vi "01.vi"() -> ()   [LabVIEW 2015]
uses:
  Libraries/LibSDL2 Wrapper/Controls/Init Flags.ctl
  Libraries/LibSDL2 Wrapper/LibSDL2.lvlib
panel:
  out "Error":string
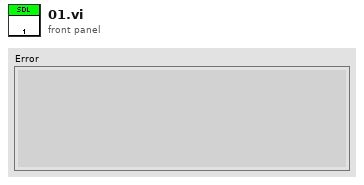
[diagram p1: front panel]
types:
  T1 = typedef "LibSDL2.lvlib/Init Flags.ctl" = u32
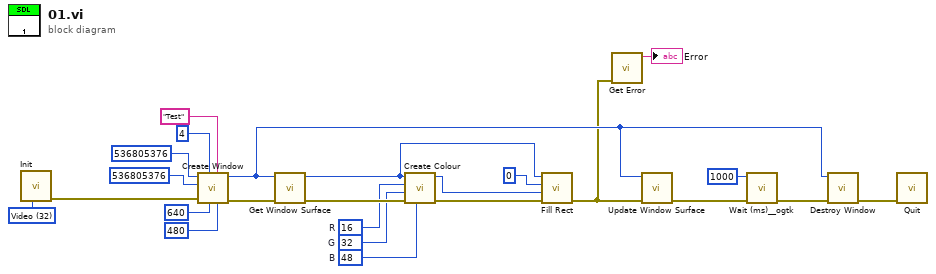
[diagram p0: block diagram]
diagram:
  w1 = u8 48  # B
  w2 = u8 32  # G
  w5 = u8 16  # R
  w24 = T1 32 items=["Timer"=1, "Audio"=16, "Video"=32, "Joystick"=512, "Haptic"=4096, "Game Controller"=8192, "Events"=16384, "No Parachute"=1048576, "Everything"=17244689] ("Init Flags")
  n1 = call "Init.vi"("Flags"=w24) -> ("error out"=w18:errorcluster)  [unwired: 9 in, 1 out]
  n2 = call "Create Window.vi"("Height"=480, "Title"="Test", "Width"=640, "Flags"=u32 4, "error in"=w18, "Position y"=u32 536805376 ("Flags"), "Position x"=u32 536805376 ("Flags")) -> ("error out"=w8:errorcluster, "Window Pointer"=w11:u32)  [unwired: 3 in]
  n3 = call "Get Window Surface.vi"("error in"=w8, "Window Pointer"=w11) -> ("error out"=w7:errorcluster, "Surface Pointer"=w10:u32)  [unwired: 8 in]
  n4 = call "Create Colour.vi"("B"=w1, "error in (no error)"=w7, "G"=w2, "R"=w5, "Surface Pointer"=w10) -> ("error out"=w6:errorcluster, "Colour"=w15:u32)  [unwired: 5 in]
  n5 = call "Fill Rect.vi"("error in (no error)"=w6, "Colour"=w15, "Rect Pointer"=u32 0, "Destination Surface Pointer"=w10) -> ("error out"=w3:errorcluster)  [unwired: 7 in]
  n6 = call "Get Error.vi"("error in"=w3) -> ("Error"=→"Error":string)  [unwired: 9 in, 1 out]
  n7 = call "Update Window Surface.vi"("error in"=w3, "Window Pointer"=w11) -> ("error out"=w14:errorcluster)  [unwired: 9 in]
  n8 = call <userlib>:"Wait (ms)__ogtk.vi"("error in (no error)"=w14, "milliseconds to wait"=u32 1000) -> ("error out"=w13:errorcluster)  [unwired: 8 in, 1 out]
  n9 = call "Destroy Window.vi"("error in"=w13, "Window Pointer"=w11) -> ("error out"=w12:errorcluster)  [unwired: 9 in]
  n10 = call "Quit.vi"("error in"=w12) -> ()  [unwired: 10 in, 1 out]
